vi "log_simple.vi"(4 "errorMsg":string="URL=", 7 "URL":string="URL=", 8 "StartTime":string, 11 "采集项":string[](array[string])) -> ()   [LabVIEW 2015]
uses:
  <vilib>/Utility/file.llb/Write Delimited Spreadsheet (string).vi
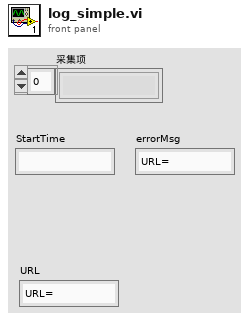
[diagram p1: front panel]
types:
  T1 = enum16{"open", "replace", "create", "open or create", "replace or create", "replace or create with confirmation"}
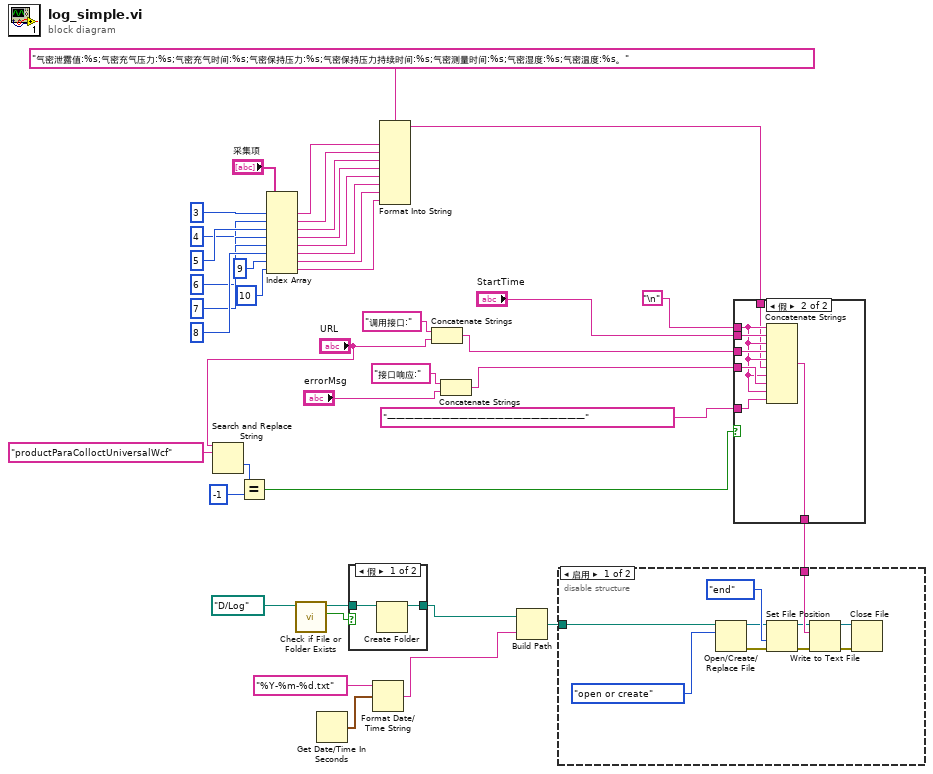
[diagram p0: block diagram]
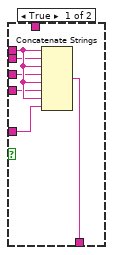
[diagram p2: hidden frame]
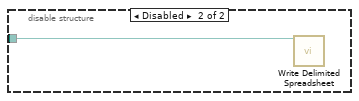
[diagram p3: hidden frame]
diagram:
  n1 = Search and Replace String(input string="URL", search string="productParaColloctUniversalWcf" ("搜索字符串")) -> (offset past replacement=w20:i32)  [unwired: 6 in, 3 out]
  n2 = Equal?(x=w20, y=-1) -> (x = y?=w19:bool)
  n3 = Index Array(array="采集项", index #1=3 ("索引"), index #2=4 ("索引"), index #3=5 ("索引"), index #4=6 ("索引"), index #5=7 ("索引"), index #6=8 ("索引"), index #7=9 ("索引"), index #8=10 ("索引")) -> (element #1=w11:string, element #2=w10:string, element #3=w9:string, element #4=w8:string, element #5=w7:string, element #6=w6:string, element #7=w2:string, element #8=w1:string)
  n4 = call <vilib>:"Check if File or Folder Exists.vi"("path"=path "D:/Log" ("路径")) -> ("file or folder exists?"=w38:bool, "dup path"=w39:path)  [unwired: 8 in, 1 out]
  n5 = Get Date/Time In Seconds() -> (seconds since 1Jan1904=w34:timestamp)
  n6 = case shown="假" w38 {
    tunnel: w39 -> [w43 w44]
    tunnel: [w42 w44] -> w36
    frame False {
      n7 = Create Folder(path (use dialog)=w43) -> (created path=w42:path)  [unwired: 2 in, 2 out]
    }
    frame True {
    }
  }
  n8 = Format Date/Time String(time format string (%c)="%Y-%m-%d.txt" ("时间格式字符串(%c)"), seconds (now)=w34) -> (date/time string=w33:string)  [unwired: 1 in]
  n9 = Format Into String(format string="气密泄露值:%s;气密充气压力:%s;气密充气时间:%s;气密保持压力:%s;气密保持压力持续时间:%s;气密测量时间:%s;气密湿度:%s;气密温度:%s。" ("value"), w11, w10, w9, w8, w7, w6, w2, w1) -> (resulting string=w5:string)  [unwired: 2 in, 1 out]
  n10 = Concatenate Strings("调用接口:" ("value"), "URL") -> (w29:string)
  n11 = Concatenate Strings("接口响应:" ("value"), "errorMsg") -> (w26:string)
  n12 = Build Path(base path=w36, name or relative path=w33) -> (appended path=w40:path)
  n13 = case shown="假" w19 {
    tunnel: [w50 w57] -> w41
    tunnel: "\n" -> [w49 w52]
    tunnel: "StartTime" -> [w48 w56]
    tunnel: w29 -> [w47 w55]
    tunnel: w26 -> [w46 w54]
    tunnel: "——————————————————————" ("value") -> [w45 w53]
    tunnel: w5 -> [_ w51]
    frame True {
      n14 = Concatenate Strings(w49, w48, w49, w47, w49, w46, w49, w45) -> (w50:string)
    }
    frame False {
      n15 = Concatenate Strings(w52, w56, w52, w55, w52, w51, w52, w54, w52, w53) -> (w57:string)
    }
  }
  n16 = disable-structure shown="启用" {
    disable-tunnel: w41 -> [w67 _]
    disable-tunnel: w40 -> [w58 w68]
    frame Enabled {
      n17 = Open/Create/Replace File(file path (use dialog)=w58, operation (0:open)=T1."open or create" ("操作(0:open)")) -> (refnum out=w62:refnum<file>, error out=w63:errorcluster)  [unwired: 4 in, 1 out]
      n18 = Set File Position(refnum=w62, from (0:start)=enum16{"start", "end", "current"}."end" ("自（0:起始）"), error in=w63) -> (refnum out=w64:refnum<file>, error out=w65:errorcluster)  [unwired: 1 in]
      n19 = Write to Text File(file (use dialog)=w64, text=w67, error in=w65) -> (refnum out=w61:refnum<file>, error out=w60:errorcluster)  [unwired: 1 in, 1 out]
      n20 = Close File(refnum=w61, error in=w60) -> ()  [unwired: 2 out]
    }
    frame Disabled {
      n21 = call-poly <vilib>:"Write Delimited Spreadsheet.vi"("file path (dialog if empty)"=w68) -> ()  [unwired: 13 in, 2 out]
    }
  }
